vi "SetControllerTemperature.vi"(11 "Temp Setpoint":dbl format="%#_13g") -> (0 "error out":errorcluster, 1 "Success?":bool)   [LabVIEW 2022 SP3]
uses:
  <vilib>/Instr/_visa.llb/VISA Configure Serial Port (Instr).vi
panel:
  in  "VISA resource name":refnum<visa-resource-name>="COM4"
  out "Returned":string
  out "Sent Command":string
  out "Temperature Setpoint Limit":i32=500
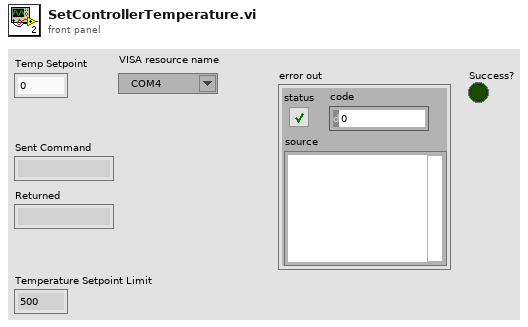
[diagram p1: front panel]
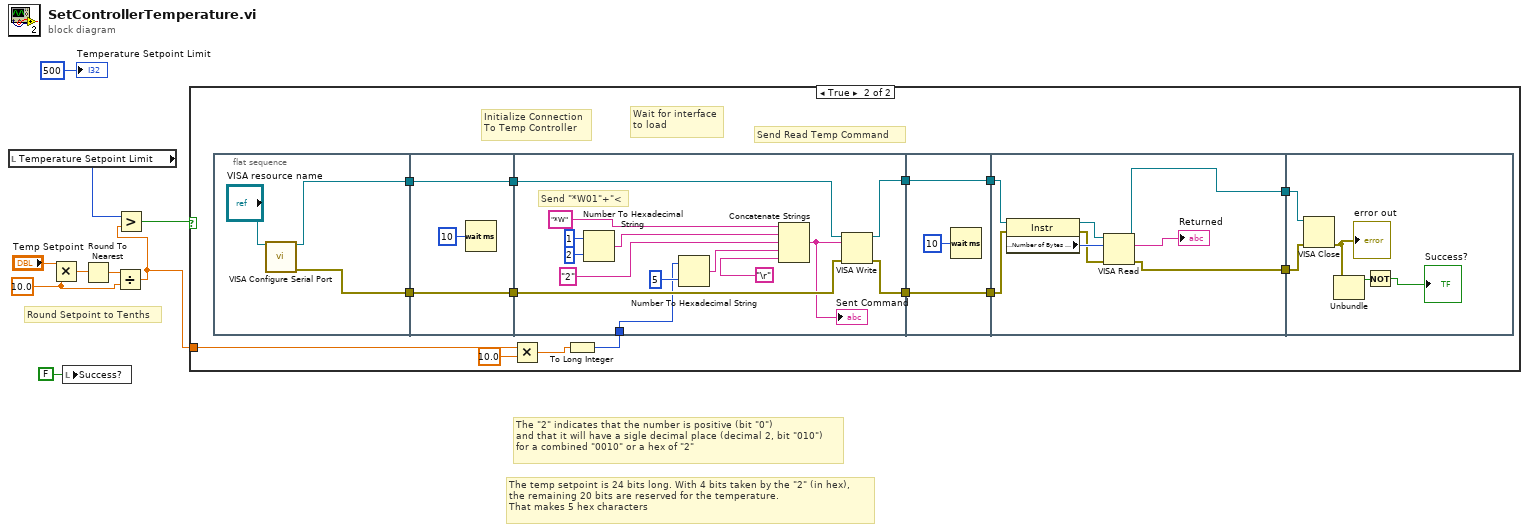
[diagram p0: block diagram]
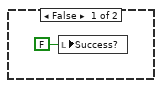
[diagram p2: hidden frame]
diagram:
  w6 = 10.0 ("y")
  # "The \"2\" indicates that the number is positive (bit \"0\")\nand that it will have a sigle decimal place (decimal 2, bit \"010\")\nfor a combined \"0010\" or a hex of \"2\""
  # "The temp setpoint is 24 bits long. With 4 bits taken by the \"2\" (in hex),\nthe remaining 20 bits are reserved for the temperature.\nThat makes 5 hex characters"
  # "Round Setpoint to Tenths"
  n1 = local read "Temperature Setpoint Limit"() -> (w4:i32)
  n2 = Multiply(x="Temp Setpoint", y=w6) -> (x*y=w8:dbl)
  n3 = local write "Success?"(FALSE ("Success?")) -> ()
  n4 = Round To Nearest(number=w8) -> (nearest integer value=w7:dbl)
  n5 = Divide(x=w7, y=w6) -> (x/y=w1:dbl)
  n6 = Greater?(x=w4, y=w1) -> (0:w3:bool)
  n7 = case shown="True" w3 {
    tunnel: w1 -> [_ w14]
    frame False {
      n8 = local write "Success?"(FALSE ("Success?")) -> ()
    }
    frame True {
      # "Initialize Connection\nTo Temp Controller"
      # "Wait for interface\nto load"
      # "Send Read Temp Command"
      n9 = flat-sequence {
        tunnel: [w27] -> w24
        tunnel: [w26] -> w23
        tunnel: w24 -> [w28]
        tunnel: w23 -> [w29]
        tunnel: [w29] -> w22
        tunnel: [w28] -> w21
        tunnel: w22 -> [w40]
        tunnel: w21 -> [w39]
        tunnel: [w38] -> w20
        tunnel: [w37] -> w19
        tunnel: w11 -> [w33]
        tunnel: w20 -> [w47]
        tunnel: w19 -> [w46]
        tunnel: [w47] -> w18
        tunnel: [w46] -> w17
        tunnel: w18 -> [w52]
        tunnel: w17 -> [w51]
        tunnel: [w50] -> w16
        tunnel: [w49] -> w15
        tunnel: w16 -> [w60]
        tunnel: w15 -> [w59]
        frame #0 {
          n10 = call-poly "VISA Configure Serial Port"("VISA resource name"="VISA resource name") -> ("VISA resource name out"=w26:refnum<visa-resource-name>, "error out"=w27:errorcluster)  [unwired: 13 in]
        }
        frame #1 {
          n11 = Wait (ms)(milliseconds to wait=u32 10) -> ()  [unwired: 1 out]
        }
        frame #2 {
          # "Send \"*W01\"+\"<"
          n12 = Number To Hexadecimal String(1:i16 2 ("width (-)"), 2:1 ("number")) -> (0:w42:string)
          n13 = Number To Hexadecimal String(1:i16 5 ("width (-)"), 2:w33) -> (0:w32:string)
          n14 = Concatenate Strings("*W" ("string to write"), w42, "2" ("string"), w32, "\r") -> (w31:string)
          "Sent Command" <- w31
          n15 = VISA Write(VISA resource name=w40, write buffer=w31, error in (no error)=w39) -> (VISA resource name out=w38:refnum<visa-resource-name>, error out=w37:errorcluster)  [unwired: 1 out]
        }
        frame #3 {
          n16 = Wait (ms)(milliseconds to wait=u32 10) -> ()  [unwired: 1 out]
        }
        frame #4 {
          n17 = property class="Instr"(reference=w52, error in=w51) -> (reference out=w53:refnum<visa-resource-name>, error out=w54:errorcluster, "Serial Settings:Number of Bytes at Serial Port"=w55:u32)
          n18 = VISA Read(VISA resource name=w53, byte count=w55, error in (no error)=w54) -> (VISA resource name out=w50:refnum<visa-resource-name>, read buffer=→"Returned":string, error out=w49:errorcluster)  [unwired: 1 out]
        }
        frame #5 {
          n19 = VISA Close(VISA resource name=w60, error in (no error)=w59) -> (error out=w58:errorcluster)
          "error out" <- w58
          n20 = Unbundle(w58) -> ("status"=w57:bool)  [unwired: 2 out]
          n21 = Not(x=w57) -> (.not. x?=→"Success?":bool)
        }
      }
      n22 = Multiply(x=w14, y=10.0) -> (x*y=w12:dbl)
      n23 = To Long Integer(number=w12) -> (32bit integer=w11:i32)
    }
  }
  "Temperature Setpoint Limit" <- 500 ("Temperature Setpoint Limit")
